vi "Get Number of Music Elements.vi"(8 "error in (no error)":errorcluster, 11 "MusicElementLibrary in":refnum<class "MusicElementLibrary.lvclass">) -> (0 "error out":errorcluster, 2 "Size":i32, 3 "MusicElementLibrary out":refnum<class "MusicElementLibrary.lvclass">)   [LabVIEW 2015, in "MusicElementLibrary.lvclass"]
uses:
  MusicElementLibrary.lvclass
  MusicElementLibrary.lvclass/MusicElementLibrary.ctl
  MusicElement.lvclass
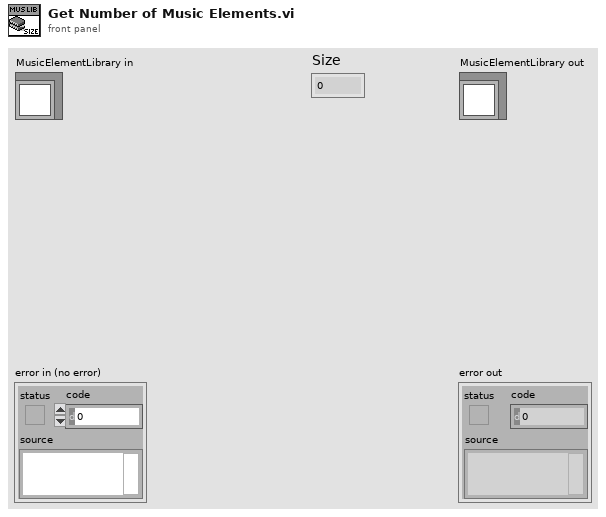
[diagram p1: front panel]
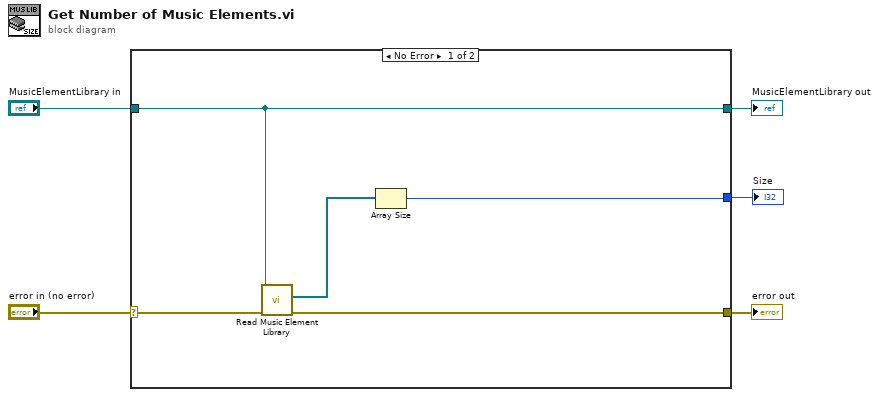
[diagram p0: block diagram]
diagram:
  n1 = case shown="No Error" "error in (no error)" {
    selector: "error in (no error)" -> [w10 w12]
    tunnel: [w9 w12] -> w4
    tunnel: [w8 w11] -> w2
    tunnel: "MusicElementLibrary in" -> [w8 w11]
    tunnel: [w6 _] -> w1
    frame No Error {
      n2 = call "Read Music Element Library.vi"("error in (no error)"=w10, "MusicElementLibrary in"=w8) -> ("error out"=w9:errorcluster, "Music Element Library"=w7:refnum<class "MusicElement.lvclass">[])  [unwired: 7 in, 1 out]
      n3 = Array Size(array=w7) -> (size(s)=w6:i32)
    }
    frame Error {
    }
  }
  "error out" <- w4
  "MusicElementLibrary out" <- w2
  "Size" <- w1
